vi "Process Command.vi"(4 "error in (no error)":errorcluster, 7 "Remote Access Commands in":refnum<class "Remote Access Commands.lvclass">) -> (0 "error out":errorcluster, 2 "Response out":T1, 3 "Remote Access Commands out":refnum<class "Remote Access Commands.lvclass">)   [LabVIEW 2015, in "Startup Processes.lvlib" / "Remote Access Commands.lvclass"]
uses:
  Remote Access Commands.lvclass
  _typedefs/JSON Response Cluster.ctl
  _typedefs/Custom Remote Access Error Codes.ctl
  Startup Processes.lvlib
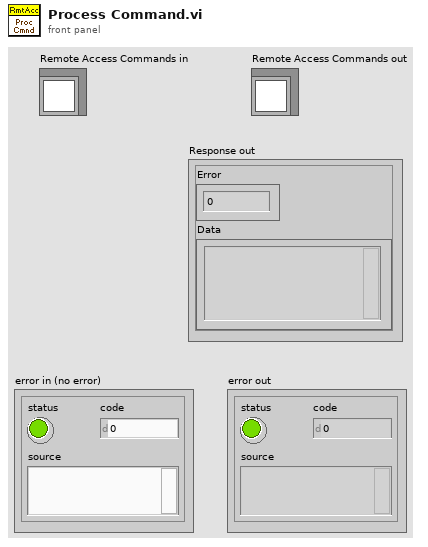
[diagram p1: front panel]
types:
  T1 = typedef "Startup Processes.lvlib/JSON Response Cluster.ctl" = cluster{"Error":i32, "Data":string}
  T2 = typedef "Startup Processes.lvlib/Custom Remote Access Error Codes.ctl" = enum16{"No Error", "CRC Error", "Update Failed"}
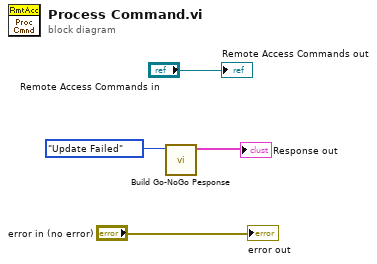
[diagram p0: block diagram]
diagram:
  n1 = call "Build Go-NoGo Pesponse.vi"("Error"=Custom_Remote_Access_Error_Codes."Update Failed") -> ("Response"=→"Response out":T1)  [unwired: 5 in, 1 out]
  "error out" <- "error in (no error)"
  "Remote Access Commands out" <- "Remote Access Commands in"
